vi "S7COMM - Format Read Request.vi"(4 "Bit Offset":u8, 6 "Read Length":u16, 7 "Variable Type":T3=enum."BIT", 8 "Data Block #":u16, 9 "Start Address":T1, 10 "Memory Area":T2 items=["P Area"=128, "I Area"=129, "O Area"=130, "M Area"=131, "DB Area"=132, "Counter"=40, "Timer"=41], 11 "S7":refnum<class "S7NetCom.lvclass">) -> (2 "S7 PDU Data":T4 format="0x%02x", 3 "S7 out":refnum<class "S7NetCom.lvclass">)   [LabVIEW 2014, in "S7NetCom.lvclass"]
doc: "____\nCopyright (c) 2019 Hampel Software Engineering (HSE), released under BSD license. More info can be found on https://dokuwiki.hampel-soft.com/code/hse/s7netcom. Original code published by Marc Christenson, Sisu Devices."
uses:
  S7NetCom.lvclass
  Controls/S7NetCom_HexByteArray.ctl
  Controls/S7NetCom_HexByte.ctl
  Controls/S7_Variable_Type.ctl
  Controls/S7_Memory_Area.ctl
  Controls/S7_Start_Address.ctl
  S7COMM - Function Codes--ring.ctl
  S7NetCom.lvclass/S7NetCom.ctl
  S7COMM - Create JOB Message Header.vi
  S7COMM - Header - Protocol ID--constant.vi
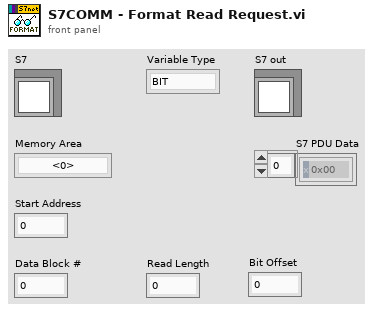
[diagram p1: front panel]
types:
  T1 = typedef "S7NetCom.lvclass/S7_Start_Address.ctl" = u16
  T2 = typedef "S7NetCom.lvclass/S7_Memory_Area.ctl" = u8
  T3 = typedef "S7NetCom.lvclass/S7_Variable_Type.ctl" = enum8{"---", "BIT", "BYTE", "CHAR", "WORD", "INT", "DWORD", "DINT", "REAL"}
  T4 = typedef "S7NetCom.lvclass/S7NetCom_HexByteArray.ctl" = T5[]
  T5 = typedef "S7NetCom.lvclass/S7NetCom_HexByte.ctl" = u8
  T6 = typedef "S7NetCom.lvclass/S7COMM - Function Codes--ring.ctl" = u8
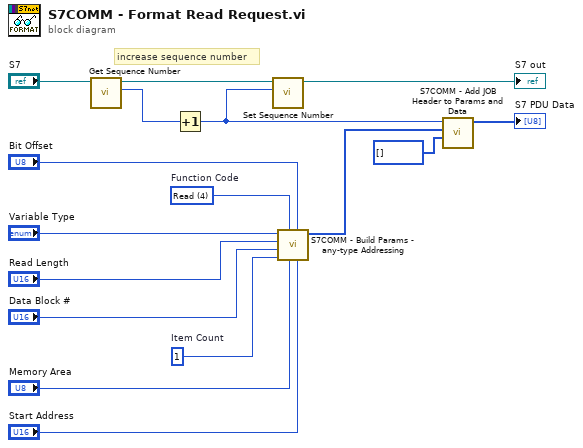
[diagram p0: block diagram]
diagram:
  w2 = u8 1  # Item Count
  w16 = T6 4 items=["Read"=4, "Write"=5]  # Function Code
  # "increase sequence number"
  n1 = call "Get Sequence Number.vi"("S7NetCom in"="S7") -> ("Sequence No."=w13:u16, "S7NetCom out"=w14:refnum<class "S7NetCom.lvclass">)  [unwired: 9 in]
  n2 = Increment(x=w13) -> (x+1=w11:u16)
  n3 = call "Set Sequence Number.vi"("Sequence No."=w11, "S7NetCom in"=w14) -> ("S7NetCom out"=→"S7 out":refnum<class "S7NetCom.lvclass">)  [unwired: 9 in]
  n4 = call "S7COMM - Build Params - any-type Addressing.vi"("Start Address"="Start Address", "Bit Offset"="Bit Offset", "S7_Memory_Area"="Memory Area", "S7_Function_Code"=w16, "Item Count"=w2, "DB Number"="Data Block #", "Count"="Read Length", "S7_Variable_Type"="Variable Type") -> ("S7 Params Byte Array"=w4:T4)  [unwired: 3 in]
  n5 = call "S7COMM - Add JOB Header to Params and Data.vi"("S7 Data"=T4 [], "S7 Parameters"=w4, "Sequence Number"=w11) -> ("S7 PDU"=→"S7 PDU Data":T4)  [unwired: 8 in]
